vi "Get VISA Resource.vi"(8 "error in (no error)":errorcluster, 11 "Thread Configuration in":refnum<class "Thread Configuration.lvclass">) -> (0 "error out":errorcluster, 2 "VISA Resource":refnum<visa-resource-name>, 3 "Thread Configuration out":refnum<class "Thread Configuration.lvclass">)   [LabVIEW 2020, in "GE Reflective Memory.lvlib" / "Thread Configuration.lvclass"]
uses:
  Thread Configuration.lvclass
  Thread Configuration.lvclass/Thread Configuration.ctl
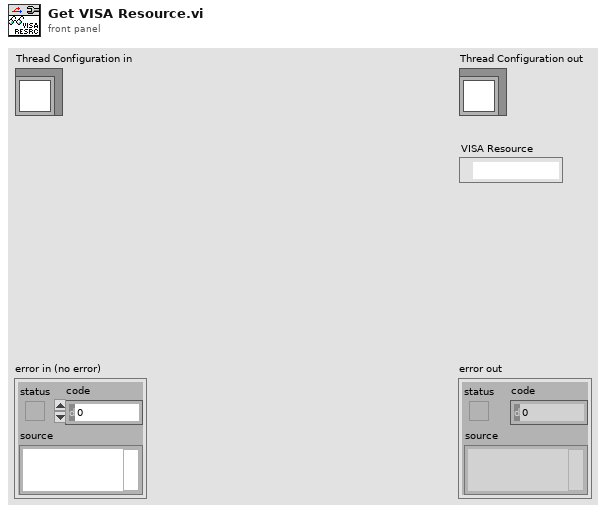
[diagram p1: front panel]
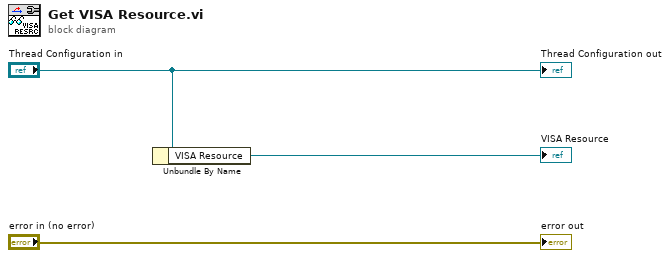
[diagram p0: block diagram]
diagram:
  n1 = Unbundle By Name("Thread Configuration in") -> ("VISA Resource"=→"VISA Resource":refnum<visa-resource-name>)
  "error out" <- "error in (no error)"
  "Thread Configuration out" <- "Thread Configuration in"
